vi "MultisitePinMapARegistered_ReserveSessionTwice_SecondReserveFails.vi"() -> (6 "pass":bool, 8 "result":string, 15 "error out":errorcluster)   [LabVIEW 2020, in "MeasurementServerTests.lvlib"]
uses:
  Runtime/MeasurementLink Pin Map Client/RPC Messages/ni_measurementlink_pinmap_v1_CreatePinMapFromXmlRequest.ctl
  Runtime/MeasurementLink Session Management Client/RPC Messages/ni_measurementlink_sessionmanagement_v1_ReserveSessionsRequest.ctl
  Runtime/MeasurementLink Session Management Client/RPC Messages/ni_measurementlink_PinMapContext.ctl
  Runtime/MeasurementLink Session Management Client/RPC Messages/ni_measurementlink_sessionmanagement_v1_ReserveAllRegisteredSessionsResponse.ctl
  Runtime/MeasurementLink Session Management Client/RPC Messages/ni_measurementlink_sessionmanagement_v1_SessionInformation.ctl
  Runtime/MeasurementLink Session Management Client/RPC Messages/nidevice_grpc_Session.ctl
  Runtime/MeasurementLink Session Management Client/RPC Messages/ni_measurementlink_sessionmanagement_v1_ChannelMapping.ctl
  Measurement Server/MeasurementServerTests.lvlib
  Runtime/MeasurementLink Session Management Client/MeasurementLink Session Management Client.lvlib
  Runtime/MeasurementLink Pin Map Client/MeasurementLink Pin Map Client.lvlib
  Runtime/MeasurementLink Discovery V1/MeasurementLink Discovery V1.lvlib
panel:
  # "Test assumes discovery service, pin map service, and session management service have already been started."
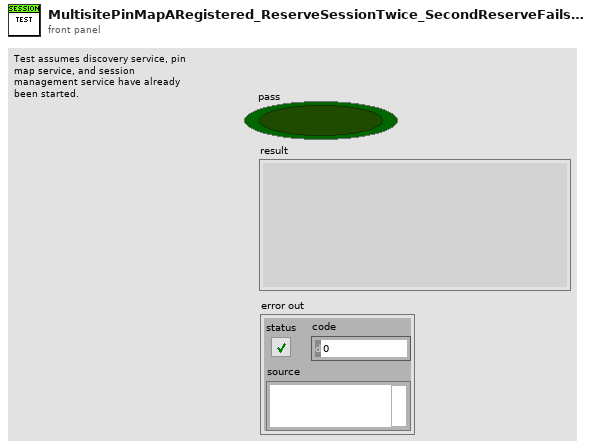
[diagram p1: front panel]
types:
  T1 = typedef "MeasurementLink Session Management Client.lvlib/ni_measurementlink_sessionmanagement_v1_ReserveAllRegisteredSessionsResponse.ctl" = cluster{"sessions":T2[]}
  T2 = typedef "MeasurementLink Session Management Client.lvlib/ni_measurementlink_sessionmanagement_v1_SessionInformation.ctl" = cluster{"session":T3, "resource_name":string, "channel_list":string, "instrument_type_id":string, "session_exists":bool, "channel_mappings":T4[]}
  T3 = typedef "MeasurementLink Session Management Client.lvlib/nidevice_grpc_Session.ctl" = cluster{"name":string}
  T4 = typedef "MeasurementLink Session Management Client.lvlib/ni_measurementlink_sessionmanagement_v1_ChannelMapping.ctl" = cluster{"pin_or_relay_name":string, "site":i32, "channel":string, "multiplexer_resource_name":string, "multiplexer_route":string}
  T5 = typedef "MeasurementLink Session Management Client.lvlib/ni_measurementlink_sessionmanagement_v1_ReserveSessionsRequest.ctl" = cluster{"pin_map_context":T6, "pin_or_relay_names":string[], "instrument_type_id":string, "timeout_in_milliseconds":i32}
  T6 = typedef "MeasurementLink Session Management Client.lvlib/ni_measurementlink_PinMapContext.ctl" = cluster{"pin_map_id":string, "sites":i32[]}
  T7 = typedef "MeasurementLink Pin Map Client.lvlib/ni_measurementlink_pinmap_v1_CreatePinMapFromXmlRequest.ctl" = cluster{"pin_map_id":string, "pin_map_xml":string}
  T8 = typedef "grpc-lvsupport-release.lvlib/grpcId.ctl" = u64
  T9 = typedef "MeasurementLink Session Management Client.lvlib/ni_measurementlink_sessionmanagement_v1_ReserveSessionsResponse.ctl" = cluster{"sessions":T2[], "multiplexer_sessions":T10[], "group_mappings":T11[]}
  T10 = typedef "MeasurementLink Session Management Client.lvlib/ni_measurementlink_sessionmanagement_v1_MultiplexerSessionInformation.ctl" = cluster{"session":T3, "resource_name":string, "multiplexer_type_id":string, "session_exists":bool}
  T11 = typedef "MeasurementLink Session Management Client.lvlib/ni_measurementlink_sessionmanagement_v1_ReserveSessionsResponse_GroupMappingsEntry.ctl" = cluster{"key":string, "value":T12}
  T12 = typedef "MeasurementLink Session Management Client.lvlib/ni_measurementlink_sessionmanagement_v1_ResolvedPinsOrRelays.ctl" = cluster{"pin_or_relay_names":string[]}
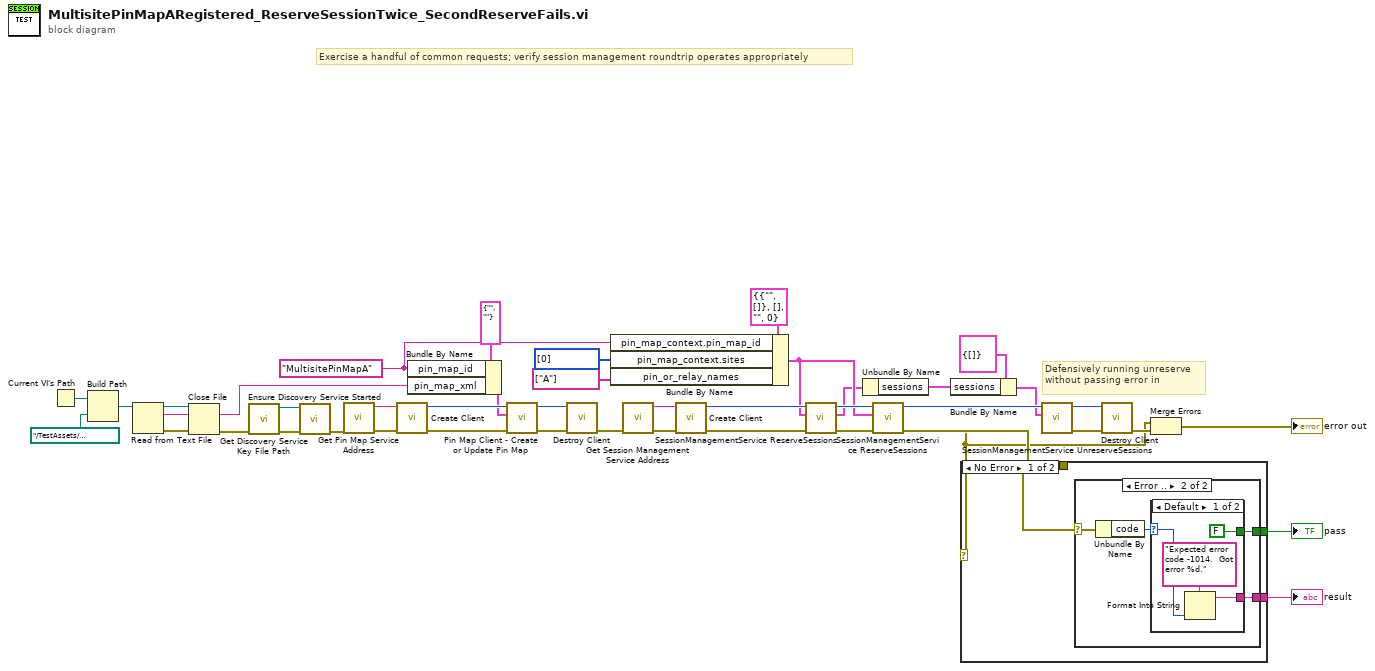
[diagram p0: block diagram]
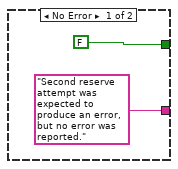
[diagram p2: hidden frame]
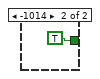
[diagram p3: hidden frame]
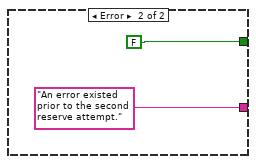
[diagram p4: hidden frame]
diagram:
  w21 = "MultisitePinMapA" ("pin_map_id")
  # "Defensively running unreserve without passing error in"
  # "Exercise a handful of common requests; verify session management roundtrip operates appropriately"
  n1 = Current VI's Path() -> (path=w37:path)
  n2 = Build Path(base path=w37, name or relative path=path "../TestAssets/MultisitePinMapA-3Instruments_3DutPins_2SystemPins_2Sites.pinmap") -> (appended path=w35:path)
  n3 = Read from Text File(file (use dialog)=w35) -> (refnum out=w31:refnum<file>, text=w33:string, error out=w32:errorcluster)  [unwired: 3 in, 1 out]
  n4 = Close File(refnum=w31, error in=w32) -> (error out=w2:errorcluster)  [unwired: 1 out]
  n5 = call "Get Discovery Service Key File Path.vi"("error in"=w2) -> ("error out"=w4:errorcluster, "key file path"=w3:path)  [unwired: 9 in]
  n6 = call "Ensure Discovery Service Started.vi"("error in"=w4, "path"=w3) -> ("error out"=w1:errorcluster)  [unwired: 8 in, 1 out]
  n7 = call "Get Pin Map Service Address.vi"("error in (no error)"=w1) -> ("error out"=w29:errorcluster, "address"=w30:string)  [unwired: 9 in]
  n8 = call "Create Client.vi"("error in"=w29, "address"=w30) -> ("error out"=w38:errorcluster, "gRPC ID Out"=w28:T8)  [unwired: 8 in]
  n9 = Bundle By Name(cluster=T7 {"pin_map_id"="", "pin_map_xml"=""} ("Request Data"), "pin_map_id"=w21, "pin_map_xml"=w33) -> (w27:T7)
  n10 = call "Pin Map Client - Create or Update Pin Map.vi"("error in (no error)"=w38, "Request Data"=w27, "gRPC ID Out"=w28) -> ("error out"=w26:errorcluster, "gRPC ID out"=w25:T8)  [unwired: 6 in, 1 out]
  n11 = call "Destroy Client.vi"("error in"=w26, "gRPC ID"=w25) -> ("error out"=w24:errorcluster)  [unwired: 9 in]
  n12 = Bundle By Name(cluster=T5 {"pin_map_context"={"pin_map_id"="", "sites"=[]}, "pin_or_relay_names"=[], "instrument_type_id"="", "timeout_in_milliseconds"=0} ("Request Data"), "pin_map_context.pin_map_id"=w21, "pin_map_context.sites"=i32[] [0], "pin_or_relay_names"=string[] ["A"]) -> (w15:T5)
  n13 = call "Get Session Management Service Address.vi"("error in (no error)"=w24) -> ("error out"=w42:errorcluster, "address"=w41:string)  [unwired: 9 in]
  n14 = call "Create Client.vi"("error in"=w42, "address"=w41) -> ("error out"=w40:errorcluster, "gRPC ID Out"=w39:T8)  [unwired: 8 in]
  n15 = call "SessionManagementService ReserveSessions.vi"("error in"=w40, "Request Data"=w15, "gRPC ID"=w39) -> ("error out"=w9:errorcluster, "Response Data"=w8:T9, "gRPC ID out"=w17:T8)  [unwired: 6 in]
  n16 = Unbundle By Name(w8) -> ("sessions"=w6:T2[])
  n17 = call "SessionManagementService ReserveSessions.vi"("error in"=w9, "Request Data"=w15, "gRPC ID"=w17) -> ("error out"=w12:errorcluster, "gRPC ID out"=w16:T8)  [unwired: 6 in, 1 out]
  n18 = Bundle By Name(cluster=T1 {"sessions"=[]} ("response data 2"), "sessions"=w6) -> (w5:T1)
  n19 = case shown="No Error" w9 {
    tunnel: [w45 FALSE] -> w14
    tunnel: [w44 "An error existed prior to the second reserve attempt." ("String")] -> w13
    tunnel: w12 -> [w43 _]
    frame No Error {
      n20 = case shown="Error .." w43 {
        selector: w43 -> [_ w51]
        tunnel: [FALSE w48] -> w45
        tunnel: ["Second reserve attempt was expected to produce an error, but no error was reported." ("String") w49] -> w44
        frame No Error {
        }
        frame Error {
          n21 = Unbundle By Name(w51) -> ("code"=w50:i32)
          n22 = case shown="Default" w50 {
            selector: w50 -> [w52 _]
            tunnel: [w54 _] -> w49
            tunnel: [FALSE TRUE] -> w48
            frame Default {
              n23 = Format Into String(format string="Expected error code -1014.  Got error %d." ("String"), w52) -> (resulting string=w54:string)  [unwired: 2 in, 1 out]
            }
            frame -1014 {
            }
          }
        }
      }
    }
    frame Error {
    }
  }
  "pass" <- w14
  "result" <- w13
  n24 = call "SessionManagementService UnreserveSessions.vi"("Request Data"=w5, "gRPC ID"=w16) -> ("error out"=w18:errorcluster, "gRPC ID out"=w23:T8)  [unwired: 7 in, 1 out]
  n25 = call "Destroy Client.vi"("error in"=w18, "gRPC ID"=w23) -> ("error out"=w11:errorcluster)  [unwired: 9 in]
  n26 = Merge Errors(w9, w11) -> (→"error out":errorcluster)
